vi "Enable Noise Cancellation.vi"(0 "VISA resource name":refnum<visa-resource-name>, 5 "Enable Noise Cancellation (F:Disable)":bool, 11 "error in (no error)":errorcluster) -> (4 "VISA resource name out":refnum<visa-resource-name>, 15 "error out":errorcluster)   [LabVIEW 2020, in "Anritsu Signal Analyzer Series.lvlib"]
doc: "Enables noice cancellation"
uses:
  Anritsu Signal Analyzer Series.lvlib
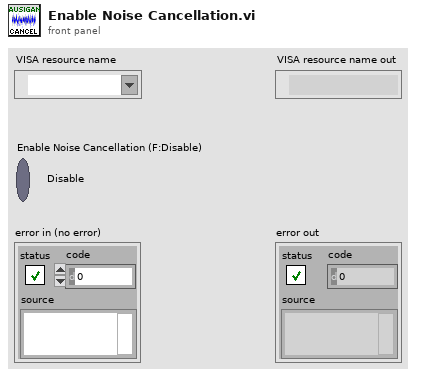
[diagram p1: front panel]
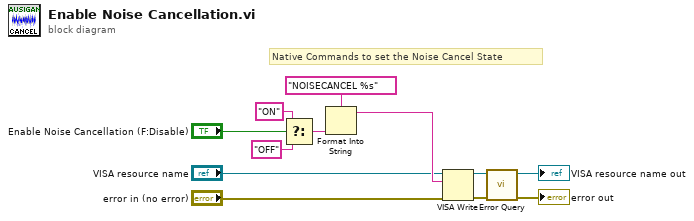
[diagram p0: block diagram]
diagram:
  # "Native Commands to set the Noise Cancel State"
  n1 = Select(t="ON" ("複数行文字列"), s="Enable Noise Cancellation (F:Disable)", f="OFF" ("複数行文字列")) -> (s? t:f=w6:string)
  n2 = Format Into String(format string="NOISECANCEL %s" ("_CommandSet"), w6) -> (resulting string=w10:string)  [unwired: 2 in, 1 out]
  n3 = VISA Write(VISA resource name="VISA resource name", write buffer=w10, error in (no error)="error in (no error)") -> (VISA resource name out=w11:refnum<visa-resource-name>, error out=w12:errorcluster)  [unwired: 1 out]
  n4 = call "Error Query.vi"("error in (no error)"=w12, "VISA resource name"=w11) -> ("error out"=→"error out":errorcluster, "VISA resource name out"=→"VISA resource name out":refnum<visa-resource-name>)  [unwired: 6 in, 2 out]
